vi "ASIC_SET_SUM_LOW.vi"(0 "connection ID":refnum<k5>, 1 "Channel":i32, 2 "Clip_sel_b":u32=1, 3 "Ib_ClipVb":u32=63, 4 "Att gain":u32, 5 "error in":errorcluster, 6 "Clip_en_b":bool=TRUE, 8 "Att_en_b":bool=TRUE) -> (11 "Data Write":string="8255@6-3_0\r\n", 13 "Register Select":string="10@5-3_0\r\n", 14 "connection ID out":refnum<k5>, 19 "error out":errorcluster)   [LabVIEW 2012]
panel:
  in  "CompBuf_en_b":bool
  in  "Action":i32=3
  out "Data":i32=8255
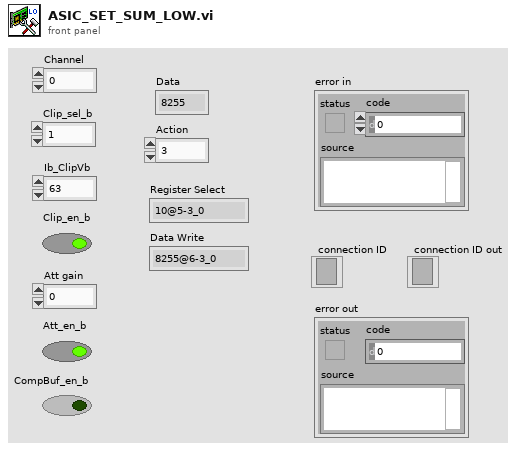
[diagram p1: front panel]
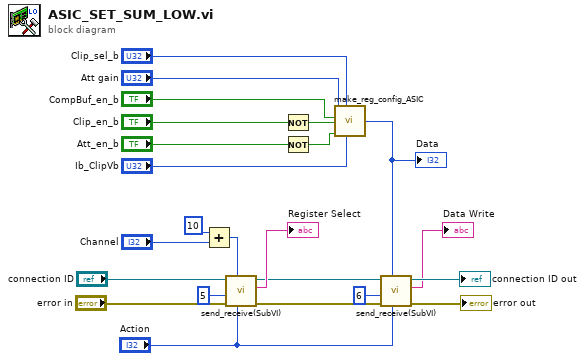
[diagram p0: block diagram]
diagram:
  n1 = Add(x=10, y="Channel") -> (x+y=w9:i32)
  n2 = call "send_receive(SubVI).vi"("Action"="Action", "Data"=w9, "error in"="error in", "Address"=5, "connection ID"="connection ID") -> ("error out"=w19:errorcluster, "connection ID out"=w5:refnum<k5>, "data in"=→"Register Select":string)  [unwired: 2 in, 2 out]
  n3 = Not(x="Clip_en_b") -> (.not. x?=w6:bool)
  n4 = Not(x="Att_en_b") -> (.not. x?=w7:bool)
  n5 = call "make_reg_config_ASIC.vi"("Ib_ClipVb"="Ib_ClipVb", "Clip_sel_b"="Clip_sel_b", "Att_en_b"=w7, "Clip_en_b"=w6, "CompBuf_en_b"="CompBuf_en_b", "Att gain"="Att gain") -> ("Out reg value"=w16:u32)
  "Data" <- w16
  n6 = call "send_receive(SubVI).vi"("Action"="Action", "Data"=w16, "error in"=w19, "Address"=6, "connection ID"=w5) -> ("error out"=→"error out":errorcluster, "connection ID out"=→"connection ID out":refnum<k5>, "data in"=→"Data Write":string)  [unwired: 2 in, 2 out]
